vi "Setmode_raw.vi"(8 "error in (no error)":errorcluster, 10 "Set_Val":u32, 11 "OneOfTemplate in":refnum<class "nixnet_grpc_DbGetDBCAttributeSizeRequest_mode_enum.lvclass">) -> (0 "error out":errorcluster, 3 "OneOfTemplate out":refnum<class "nixnet_grpc_DbGetDBCAttributeSizeRequest_mode_enum.lvclass">)   [LabVIEW 2019, in "grpc-xnet_client.lvlib" / "nixnet_grpc_DbGetDBCAttributeSizeRequest_mode_enum.lvclass"]
uses:
  nixnet_grpc_DbGetDBCAttributeSizeRequest_mode_enum.lvclass
  nixnet_grpc_DbGetDBCAttributeSizeRequest_mode_enum.lvclass/nixnet_grpc_DbGetDBCAttributeSizeRequest_mode_enum.ctl
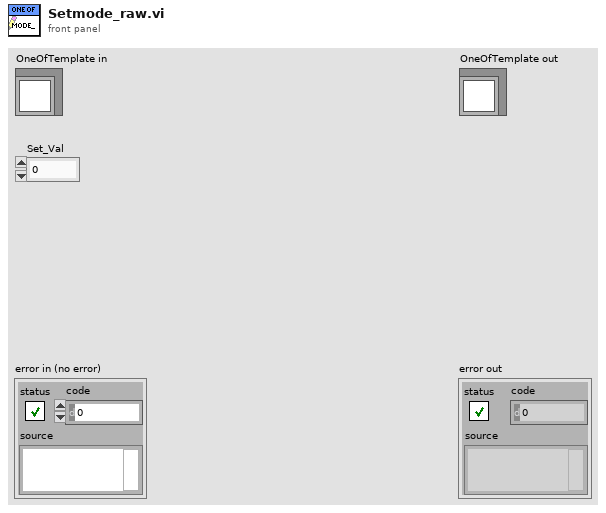
[diagram p1: front panel]
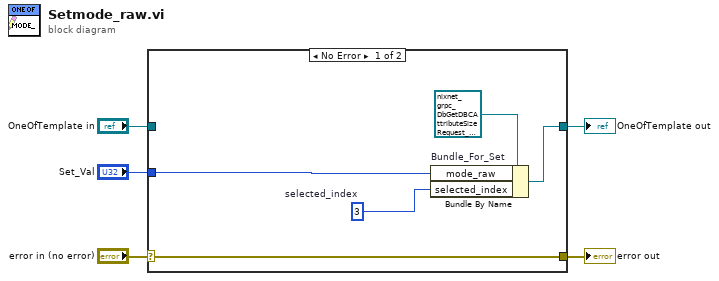
[diagram p0: block diagram]
diagram:
  n1 = case shown="No Error" "error in (no error)" {
    selector: "error in (no error)" -> [w10 w11]
    tunnel: [w10 w11] -> w4
    tunnel: [w9 w12] -> w2
    tunnel: "OneOfTemplate in" -> [_ w12]
    tunnel: "Set_Val" -> [w8 _]
    frame No Error {
      w7 = 3  # selected_index
      n2 = Bundle By Name "Bundle_For_Set"(cluster=refnum<class "nixnet_grpc_DbGetDBCAttributeSizeRequest_mode_enum.lvclass"> refnum ("OneOfTemplate in"), "mode_raw"=w8, "selected_index"=w7) -> (w9:refnum<class "nixnet_grpc_DbGetDBCAttributeSizeRequest_mode_enum.lvclass">)
    }
    frame Error {
    }
  }
  "error out" <- w4
  "OneOfTemplate out" <- w2
